vi "Configure CAN Trigger Source.vi"(0 "VISA resource name":refnum<visa-resource-name>, 1 "Trigger (0: SOF)":u16(ring) items=["SOF", "Data", "Error", "IDData", "IDEither", "IDRemote"], 5 "Trigger Source (0: Channel 1)":u16(ring) items=["Channel 1", "Channel 2", "Channel 3", "Channel 4", "DIG 0", "DIG 1", "DIG 2", "DIG 3", "DIG 4", "DIG 5", "DIG 6", "DIG 7", "DIG 8", "DIG 9", "DIG 10", "DIG 11", "DIG 12", "DIG 13", "DIG 14", "DIG 15", "EXT"], 9 "Signal (0: Rx)":u16(ring) items=["RX", "TX", "CAN_H", "CAN_L", "Differential"], 11 "error in (no error)":errorcluster, 12 "Baud Rate (11: 1 000 000)":u16(ring)=11 items=["10 000", "20 000", "33 300", "50 000", "62 500", "83 300", "100 000", "125 000", "250 000", "500 000", "800 000", "1 000 000"]) -> (4 "VISA resource name out":refnum<visa-resource-name>, 15 "error out":errorcluster)   [LabVIEW 2017, in "Agilent 6000 Series.lvlib"]
doc: "This VI configures the CAN trigger. \n\n<B>NOTE:</B>\n\nThis VI is only valid for 6000 Series models. An error will be thrown if this VI is run with 5000 Series scopes."
uses:
  <instrlib>/Agilent 6000 Series/Agilent 6000 Series.lvlib
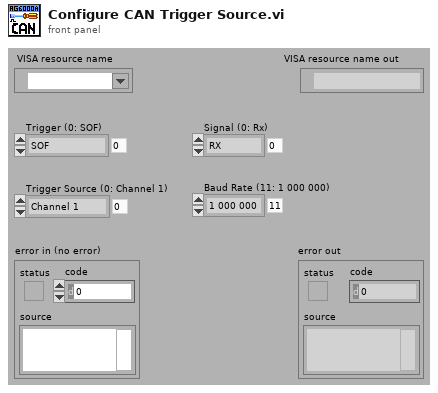
[diagram p1: front panel]
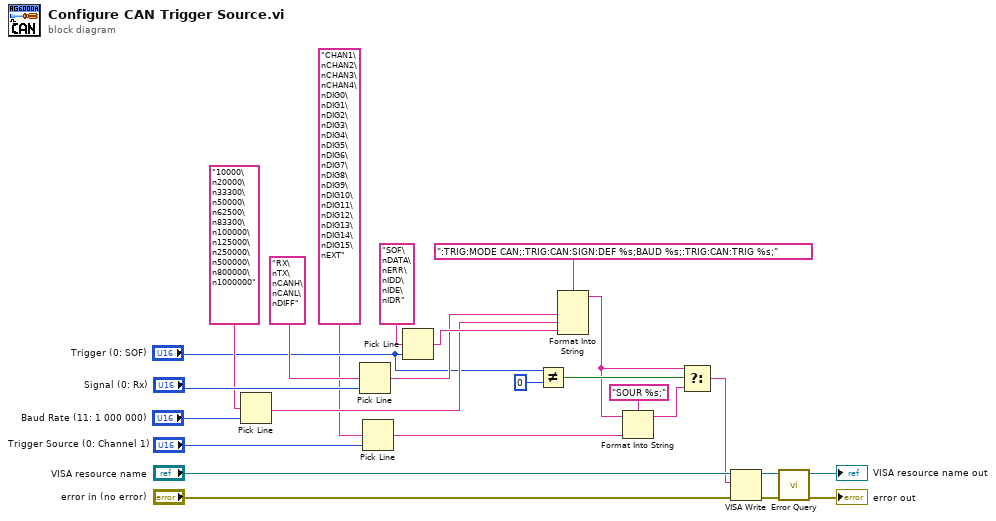
[diagram p0: block diagram]
diagram:
  n1 = Pick Line(multi-line string="10000\n20000\n33300\n50000\n62500\n83300\n100000\n125000\n250000\n500000\n800000\n1000000", line index="Baud Rate (11: 1 000 000)") -> (output string=w12:string)  [unwired: 1 in]
  n2 = Pick Line(multi-line string="RX\nTX\nCANH\nCANL\nDIFF", line index="Signal (0: Rx)") -> (output string=w11:string)  [unwired: 1 in]
  n3 = Pick Line(multi-line string="CHAN1\nCHAN2\nCHAN3\nCHAN4\nDIG0\nDIG1\nDIG2\nDIG3\nDIG4\nDIG5\nDIG6\nDIG7\nDIG8\nDIG9\nDIG10\nDIG11\nDIG12\nDIG13\nDIG14\nDIG15\nEXT", line index="Trigger Source (0: Channel 1)") -> (output string=w5:string)  [unwired: 1 in]
  n4 = Pick Line(multi-line string="SOF\nDATA\nERR\nIDD\nIDE\nIDR", line index="Trigger (0: SOF)") -> (output string=w15:string)  [unwired: 1 in]
  n5 = Not Equal?(x="Trigger (0: SOF)", y=u16 0) -> (x != y?=w8:bool)
  n6 = Format Into String(format string=":TRIG:MODE CAN;:TRIG:CAN:SIGN:DEF %s;BAUD %s;:TRIG:CAN:TRIG %s;" ("Source Command"), w11, w12, w15) -> (resulting string=w6:string)  [unwired: 2 in, 1 out]
  n7 = Format Into String(format string="SOUR %s;", initial string=w6, w5) -> (resulting string=w4:string)  [unwired: 1 in, 1 out]
  n8 = Select(t=w6, s=w8, f=w4) -> (s? t:f=w3:string)
  n9 = VISA Write(VISA resource name="VISA resource name", write buffer=w3, error in (no error)="error in (no error)") -> (VISA resource name out=w21:refnum<visa-resource-name>, error out=w20:errorcluster)  [unwired: 1 out]
  n10 = call <instrlib>:"Error Query.vi"("error in (no error)"=w20, "VISA resource name"=w21) -> ("error out"=→"error out":errorcluster, "VISA resource name out"=→"VISA resource name out":refnum<visa-resource-name>)  [unwired: 6 in, 2 out]
